vi "empty buffer check.vi"(10 "Full?":bool, 11 "Index":i32) -> (3 "empty buffer?":bool)   [LabVIEW 2021, in "Ring Buffer Time Series Data.lvlib"]
uses:
  Ring Buffer Time Series Data.lvlib
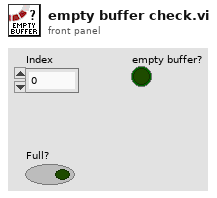
[diagram p1: front panel]
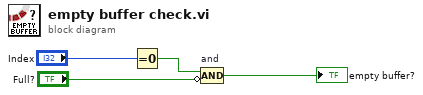
[diagram p0: block diagram]
diagram:
  n1 = Equal To 0?(x="Index") -> (x = 0?=w4:bool)
  n2 = Compound Arithmetic op=AND "and"(w4, invert "Full?") -> (→"empty buffer?":bool)
